vi "Bscaling.vi"() -> ()   [LabVIEW 2020]
panel:
  out "2plots":cluster{dbl[], dbl[]}[](graph)
  in  "24.6V":cluster{dbl[], dbl[]}[](graph)=[{array[8344 elements], array[8344 elements]}]
  in  "25V":cluster{dbl[], dbl[]}[](graph)=[{array[8344 elements], array[8344 elements]}]
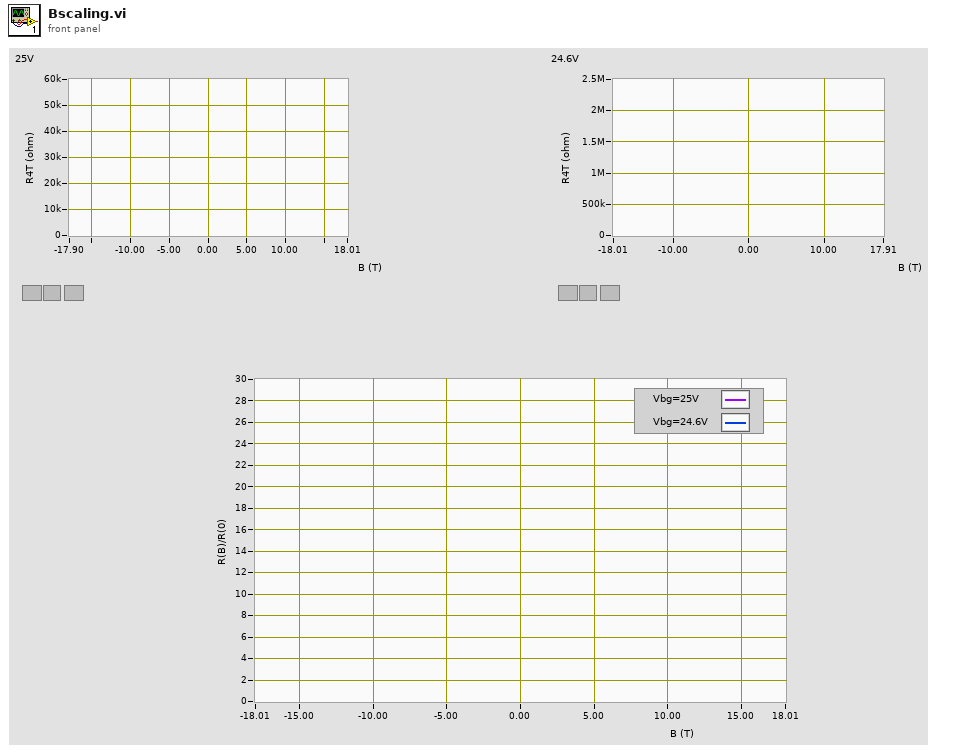
[diagram p1: front panel]
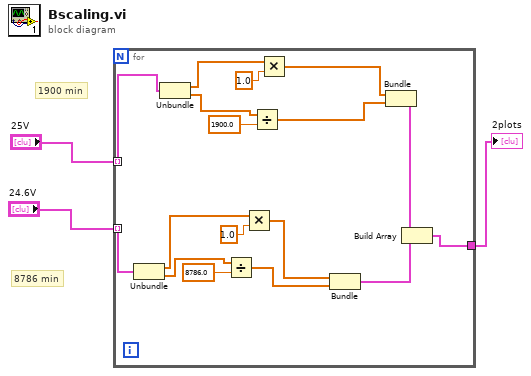
[diagram p0: block diagram]
diagram:
  # "8786 min"
  # "1900 min"
  n1 = for {
    tunnel: "25V" -> [w18] mode=indexing
    tunnel: "24.6V" -> [w13] mode=indexing
    tunnel: [w20] -> w3
    n2 = Unbundle(w13) -> (w4:dbl[], w15:dbl[])
    n3 = Unbundle(w18) -> (w9:dbl[], w17:dbl[])
    n4 = Divide(x=w15, y=8786.0) -> (x/y=w10:dbl[])
    n5 = Multiply(x=w4, y=1.0) -> (x*y=w5:dbl[])
    n6 = Divide(x=w17, y=1900.0) -> (x/y=w11:dbl[])
    n7 = Multiply(x=w9, y=1.0) -> (x*y=w8:dbl[])
    n8 = Bundle(w5, w10) -> (w12:cluster{dbl[], dbl[]})  [unwired: 1 in]
    n9 = Bundle(w8, w11) -> (w16:cluster{dbl[], dbl[]})  [unwired: 1 in]
    n10 = Build Array(w16, w12) -> (w20:cluster{dbl[], dbl[]}[])
  }
  "2plots" <- w3
